vi "Get Steering Frame Velocity from Motors.vi"(6 "ccw caster motor velocity states":dbl[](array[numeric]), 7 "wheel indexes":i32[](array[numeric]), 8 "error in (no error)":errorcluster, 9 "ccw motor angle states (rad)":dbl[](array[numeric]), 10 "ccw motor velocity states":dbl[](array[numeric]), 11 "steering frame in":refnum<class "NI_Robotics_Steering Frame.lvclass">) -> (0 "error out":errorcluster, 2 "estimated steering frame velocity":dbl[](array[numeric]), 3 "steering frame out":refnum<class "NI_Robotics_Steering Frame.lvclass">)   [LabVIEW 2017, in "NI_Robotics_Steering Frame.lvclass"]
doc: "Calculates the steering frame velocity or arc velocity required to best satisfy the velocity and angle of each motor. You must manually select the polymorphic instance to use."
uses:
  <vilib>/robotics/Steering/Steering Frame/NI_Robotics_Steering Frame.lvclass
  <vilib>/robotics/Steering/Steering Frame/NI_Robotics_Steering Frame.lvclass/NI_Robotics_Steering Frame.ctl
  <vilib>/robotics/Utilities/Generate Error.vi
  <vilib>/robotics/Steering/Steering Frame/Merge Wheel States.vi
  <vilib>/robotics/Steering/Wheel/Read Wheel State from Motors.vi
  <vilib>/robotics/Steering/Wheel/Create Wheel Angular Velocity Row_Frame.vi
  <vilib>/robotics/Steering/Wheel/Create Caster Angular Velocity Row_Frame.vi
  <vilib>/robotics/Steering/Wheel/Set Current Caster Angle_Frame.vi
  <vilib>/robotics/Steering/Wheel/Update Motor Velocity State_Frame.vi
  <vilib>/robotics/Steering/Wheel/Update Steering Motor Angle State_Frame.vi
  <vilib>/robotics/Steering/Wheel/Update Caster Motor Velocity State_Frame.vi
  <vilib>/Analysis/7linalg.llb/Solve General Linear Equations with SVD (DBL).vi
  <vilib>/robotics/Steering/Wheel/Update Motor Velocity State.vi
  <vilib>/robotics/Steering/Wheel/NI_Robotics_Wheel.lvclass
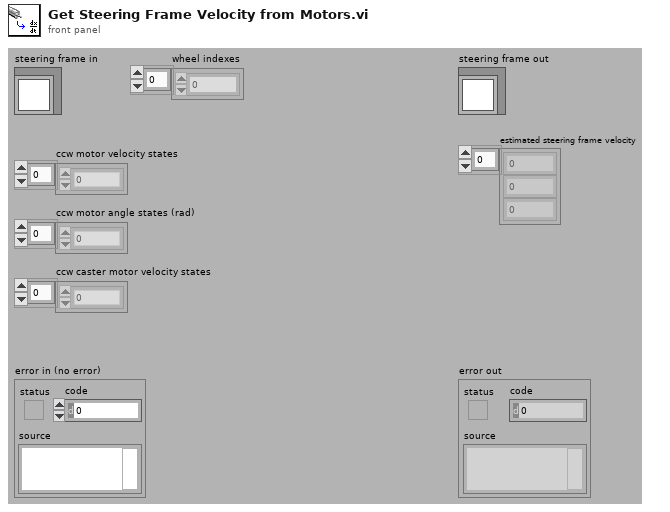
[diagram p1: front panel]
types:
  T1 = cluster{"wheel index (all)":i32, "wheel index (used)":i32, "wheels used":i32}
  T2 = typedef "NI_Matrix.lvlib/RealMatrix.ctl" = dbl[][]
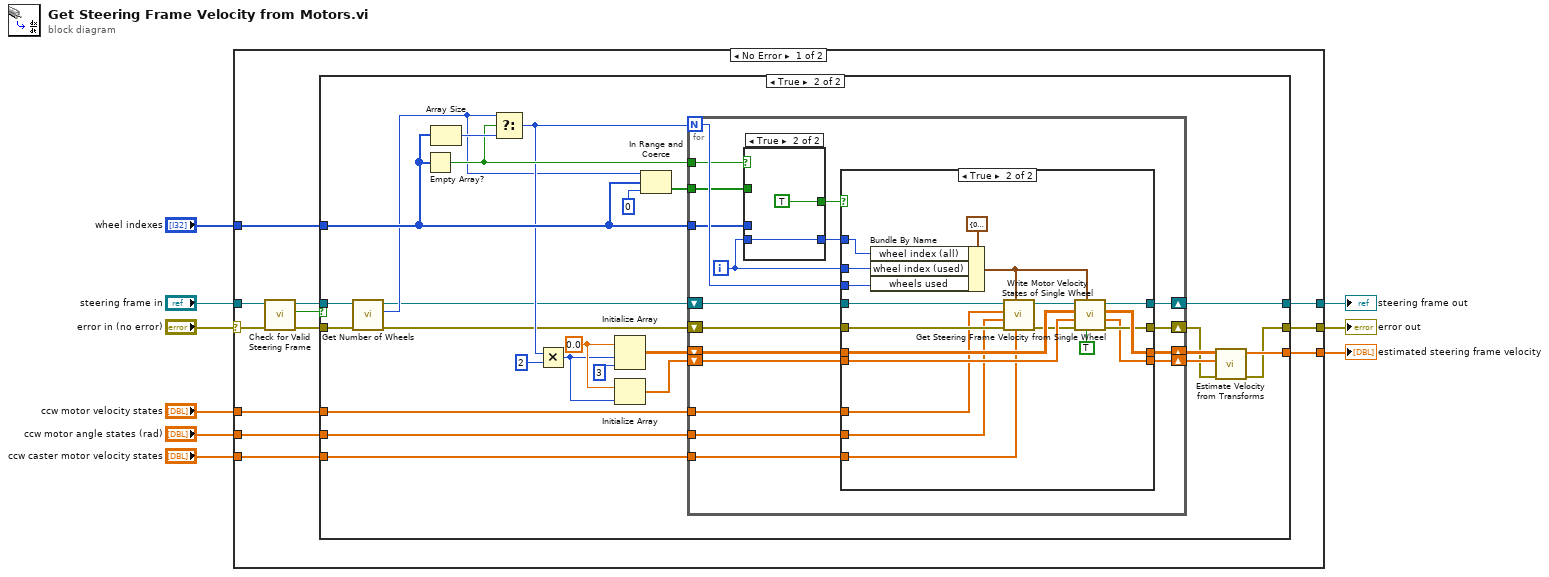
[diagram p0: block diagram]
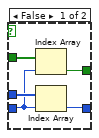
[diagram p4: hidden frame]
diagram:
  n1 = case shown="No Error" "error in (no error)" {
    selector: "error in (no error)" -> [w16 w99]
    tunnel: [w20 w99] -> w5
    tunnel: [w19 w98] -> w6
    tunnel: "steering frame in" -> [w18 w98]
    tunnel: [w21 _] -> w4
    tunnel: "wheel indexes" -> [w13 _]
    tunnel: "ccw motor velocity states" -> [w12 _]
    tunnel: "ccw motor angle states (rad)" -> [w11 _]
    tunnel: "ccw caster motor velocity states" -> [w10 _]
    frame No Error {
      n2 = call <vilib>:"Check for Valid Steering Frame.vi"("error in (no error)"=w16, "steering frame in"=w18) -> ("error out"=w15:errorcluster, "valid?"=w14:bool, "steering frame out"=w17:refnum<class "NI_Robotics_Steering Frame.lvclass">)  [unwired: 7 in]
      n3 = case shown="True" w14 {
        tunnel: [_ w26] -> w21
        tunnel: [w22 w25] -> w20
        tunnel: [w23 w48] -> w19
        tunnel: w17 -> [w23 w35]
        tunnel: w15 -> [w22 w33]
        tunnel: w13 -> [_ w49]
        tunnel: w12 -> [_ w31]
        tunnel: w11 -> [_ w30]
        tunnel: w10 -> [_ w29]
        frame False {
        }
        frame True {
          w39 = 0.0 ("element")
          n4 = call <vilib>:"Get Number of Wheels.vi"("error in (no error)"=w33, "steering frame in"=w35) -> ("error out"=w32:errorcluster, "number of wheels"=w36:i32, "steering frame out"=w34:refnum<class "NI_Robotics_Steering Frame.lvclass">)  [unwired: 7 in]
          n5 = Empty Array?(array=w49) -> (empty?=w44:bool)
          n6 = Array Size(array=w49) -> (size(s)=w47:i32)
          n7 = Select(t=w36, s=w44, f=w47) -> (s? t:f=w43:i32)
          n8 = Multiply(x=w43, y=2) -> (x*y=w38:i32)
          n9 = Initialize Array(w39, w38, 3 ("dimension size")) -> (w40:dbl[][])
          n10 = Initialize Array(w39, w38) -> (w37:dbl[])
          n11 = In Range and Coerce(upper limit=w36, x=w49, lower limit=0) -> (In Range?=w45:bool[])  [unwired: 1 out]
          n12 = for {
            N: w43 -> [w61]
            shift-right: [w62] -> w28
            shift-left: w40 -> [w63]
            shift-right: [w67] -> w24
            shift-left: w32 -> [w66]
            shift-right: [w64] -> w27
            shift-left: w37 -> [w65]
            tunnel: w49 -> [w60]
            tunnel: w45 -> [w59]
            tunnel: w44 -> [w56]
            shift-right: [w54] -> w48
            shift-left: w34 -> [w55]
            tunnel: w31 -> [w52]
            tunnel: w30 -> [w51]
            tunnel: w29 -> [w50]
            i -> [w53]
            n13 = case shown="True" w56 {
              tunnel: w60 -> [w95 _]
              tunnel: w53 -> [w93 w97]
              tunnel: [w92 w97] -> w58
              tunnel: w59 -> [w94 _]
              tunnel: [w91 TRUE ("lower limit")] -> w57
              frame False {
                n14 = Index Array(array=w94, index=w93) -> (element=w91:bool)
                n15 = Index Array(array=w95, index=w93) -> (element=w92:i32)
              }
              frame True {
              }
            }
            n16 = case shown="True" w57 {
              tunnel: [w68 w87] -> w67
              tunnel: w66 -> [w68 w77]
              tunnel: w65 -> [w69 w88]
              tunnel: [w69 w86] -> w64
              tunnel: w63 -> [w71 w90]
              tunnel: [w71 w89] -> w62
              tunnel: w61 -> [_ w81]
              tunnel: w58 -> [_ w83]
              tunnel: w55 -> [w70 w79]
              tunnel: [w70 w85] -> w54
              tunnel: w53 -> [_ w82]
              tunnel: w52 -> [_ w74]
              tunnel: w51 -> [_ w73]
              tunnel: w50 -> [_ w72]
              frame False {
              }
              frame True {
                n17 = Bundle By Name(cluster=T1 {"wheel index (all)"=0, "wheel index (used)"=0, "wheels used"=0} ("index info"), "wheel index (all)"=w83, "wheel index (used)"=w82, "wheels used"=w81) -> (w75:T1)
                n18 = call <vilib>:"Write Motor Velocity States of Single Wheel.vi"("ccw caster motor velocity states"=w72, "index info"=w75, "error in (no error)"=w77, "ccw motor angle states (rad)"=w73, "ccw motor velocity states"=w74, "steering frame in"=w79) -> ("error out"=w76:errorcluster, "steering frame out"=w78:refnum<class "NI_Robotics_Steering Frame.lvclass">)  [unwired: 4 in]
                n19 = call <vilib>:"Get Steering Frame Velocity from Single Wheel.vi"("get motor data"=TRUE, "index info"=w75, "error in (no error)"=w76, "velocity transform vector in"=w88, "velocity transform matrix in"=w90, "steering frame in"=w78) -> ("error out"=w87:errorcluster, "velocity transform vector out"=w86:dbl[], "velocity transform matrix out"=w89:T2, "steering frame out"=w85:refnum<class "NI_Robotics_Steering Frame.lvclass">)  [unwired: 2 in]
              }
            }
          }
          n20 = call <vilib>:"Estimate Velocity from Transforms.vi"("error in (no error)"=w24, "velocity transform vector in"=w27, "velocity transform matrix in"=w28) -> ("error out"=w25:errorcluster, "estimated steering frame velocity"=w26:dbl[])  [unwired: 7 in]
        }
      }
    }
    frame Error {
    }
  }
  "error out" <- w5
  "steering frame out" <- w6
  "estimated steering frame velocity" <- w4
